vi "Insert Scheduled Transfer Handles.vi"(4 "Label in":T1 {"Words"."Param Setting"."Num Bits" min=1 max=32; "Words"."Param Setting"."Start Bit" min=8 max=31; "Words"."Block Data Refs"."Data Reference" format="%.0x"; "Label" format="%.0o"}, 7 "Tx channel handle in":u32, 8 "error in (no error)":errorcluster) -> (0 "error out":errorcluster, 3 "Label out":T1 {"Words"."Param Setting"."Num Bits" min=1 max=32; "Words"."Param Setting"."Start Bit" min=8 max=31; "Words"."Block Data Refs"."Data Reference" format="%.0x"; "Label" format="%.0o"})   [LabVIEW 2016, in "Ballard Arinc-429 Engine.lvlib"]
uses:
  Ballard Arinc-429 Engine.lvlib
  RT Controls/RT Label Settings.ctl
  Shared/Controls and Global/Label.ctl
  Shared/Controls and Global/transferPeriod.ctl
  RT Controls/Driver Data.ctl
  RT Controls/RT Word Settings.ctl
  <vilib>/NI Veristand/Custom Device API/Block Data Reference.ctl
  <vilib>/NI Veristand/Custom Device API/Data Reference.ctl
  RT Controls/RT Param Setting.ctl
  Shared/Controls and Global/Start Bit.ctl
  Shared/Controls and Global/Number of Bits.ctl
  Shared/Controls and Global/TransferType.ctl
  <instrlib>/AIT 429/AIT 429.lvlib
  Shared/Ballard Arinc-429 Shared.lvlib
  <vilib>/NI Veristand/Custom Device API/Custom Device API.lvlib
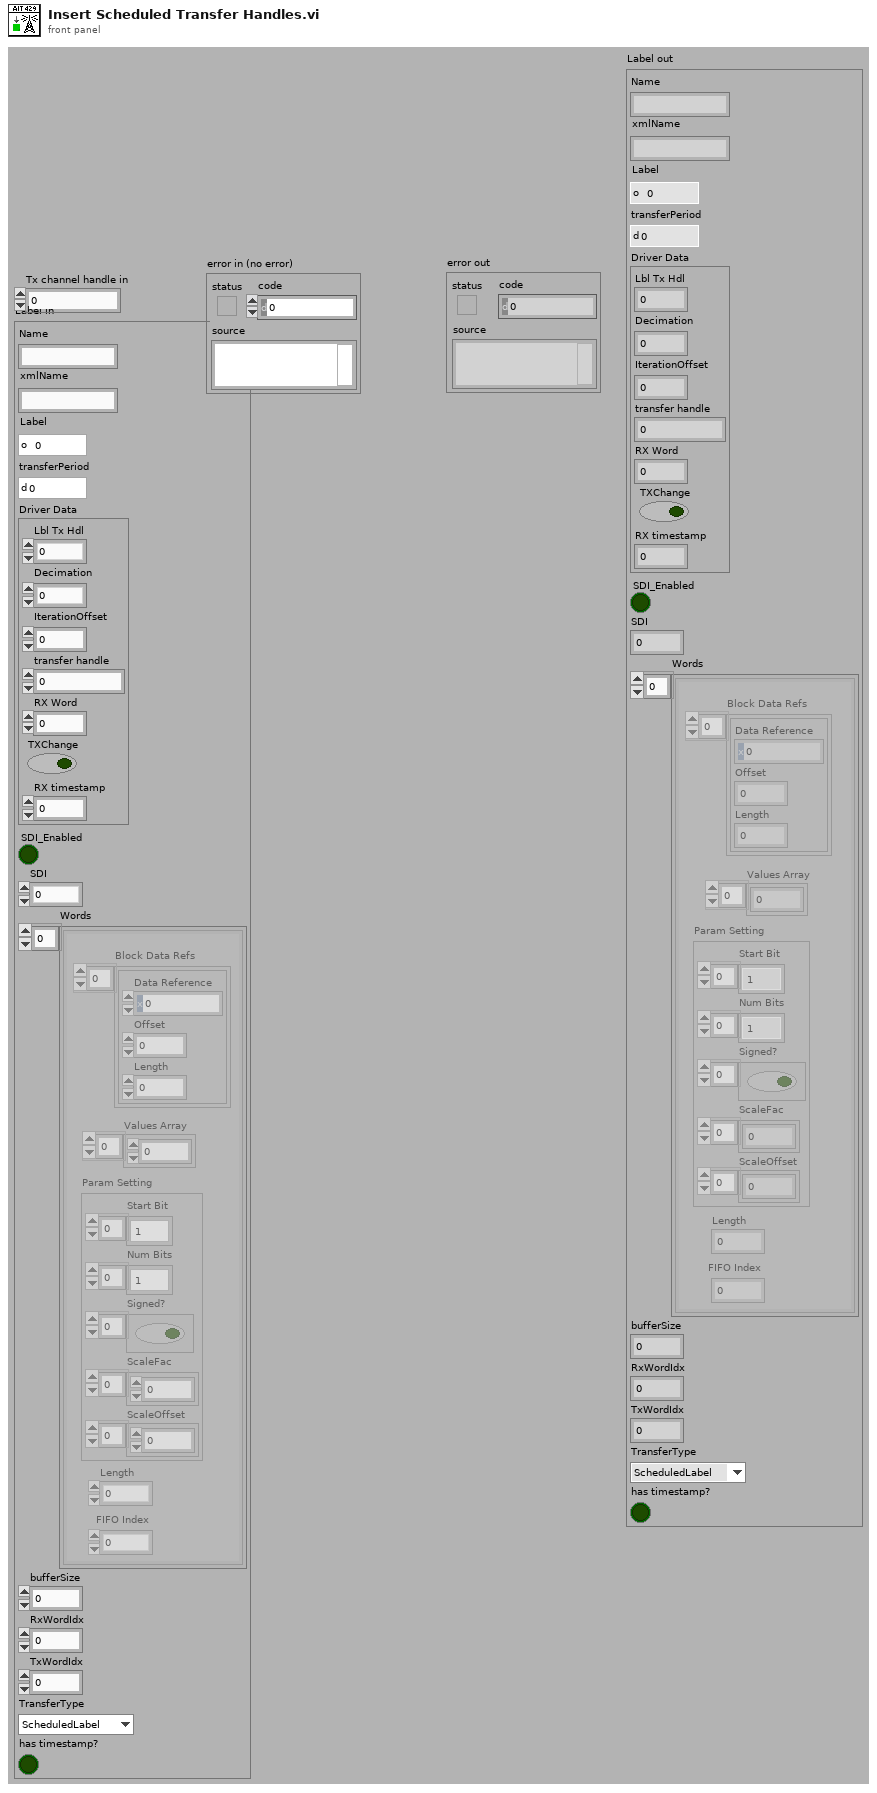
[diagram p1: front panel]
types:
  T1 = typedef "Ballard Arinc-429 Engine.lvlib/RT Label Settings.ctl" = cluster{"Name":string, "xmlName":string, "Label":T2, "transferPeriod":T3, "Driver Data":T4, "SDI_Enabled":bool, "SDI":u8, "Words":T5[], "bufferSize":u32, "RxWordIdx":i32, "TxWordIdx":i32, "TransferType":T11, "has timestamp?":bool}
  T2 = typedef "Ballard Arinc-429 Shared.lvlib/Label.ctl" = u8
  T3 = typedef "Ballard Arinc-429 Shared.lvlib/transferPeriod.ctl" = u32
  T4 = typedef "Ballard Arinc-429 Engine.lvlib/Driver Data.ctl" = cluster{"Lbl Tx Hdl":u32, "Decimation":i32, "IterationOffset":i32, "transfer handle":u32, "RX Word":u32, "TXChange":bool, "RX timestamp":dbl}
  T5 = typedef "Ballard Arinc-429 Engine.lvlib/RT Word Settings.ctl" = cluster{"Block Data Refs":T6[], "Values Array":dbl[], "Length":i32, "FIFO Index":i32, "Param Setting":T8}
  T6 = typedef "Custom Device API.lvlib/Block Data Reference.ctl" = cluster{"Data Reference":T7, "Offset":u64, "Length":u64}
  T7 = typedef "Custom Device API.lvlib/Data Reference.ctl" = i32
  T8 = typedef "Ballard Arinc-429 Engine.lvlib/RT Param Setting.ctl" = cluster{"Start Bit":T9[], "Num Bits":T10[], "Signed?":bool[], "ScaleFac":dbl[], "ScaleOffset":dbl[]}
  T9 = typedef "Ballard Arinc-429 Shared.lvlib/Start Bit.ctl" = i32
  T10 = typedef "Ballard Arinc-429 Shared.lvlib/Number of Bits.ctl" = i32
  T11 = typedef "Ballard Arinc-429 Shared.lvlib/TransferType.ctl" = enum16{"ScheduledLabel", "Acyclic", "Block", "Strobe"}
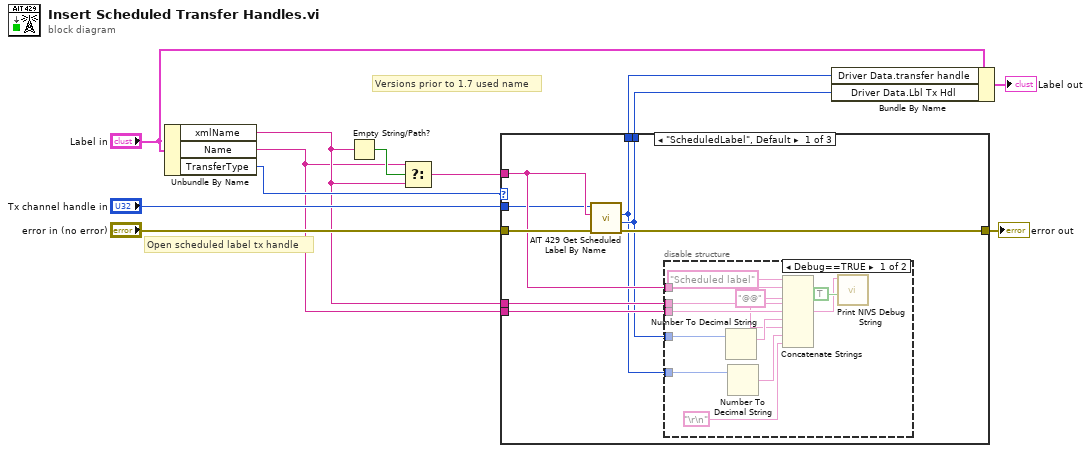
[diagram p0: block diagram]
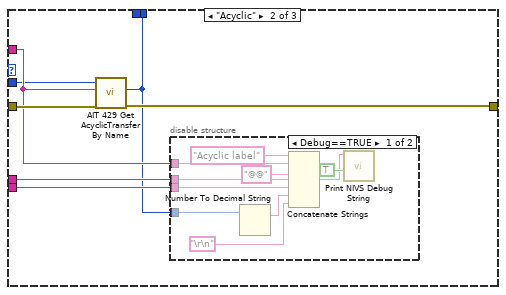
[diagram p3: hidden frame]
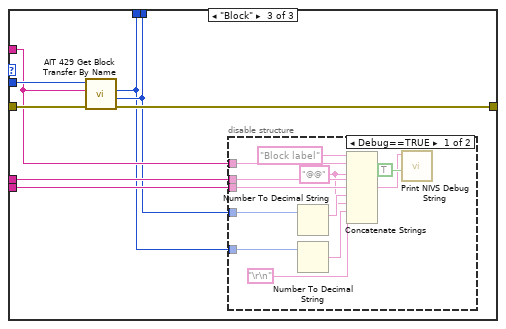
[diagram p5: hidden frame]
diagram:
  # "Open scheduled label tx handle"
  # "Versions prior to 1.7 used name"
  n1 = Unbundle By Name("Label in") -> ("xmlName"=w2:string, "Name"=w1:string, "TransferType"=w3:T11)
  n2 = Empty String/Path?(string/path=w2) -> (empty?=w5:bool)
  n3 = Select(t=w1, s=w5, f=w2) -> (s? t:f=w4:string)
  n4 = case shown="\"ScheduledLabel\", Default" w3 {
    tunnel: "error in (no error)" -> [w20 w39 w57]
    tunnel: [w14 w33 w51] -> w9
    tunnel: [w13 _ w50] -> w8
    tunnel: "Tx channel handle in" -> [w15 w34 w53]
    tunnel: [w19 w38 w56] -> w6
    tunnel: w4 -> [w18 w35 w52]
    tunnel: w2 -> [w17 w37 w55]
    tunnel: w1 -> [w16 w36 w54]
    frame "ScheduledLabel", Default {
      n5 = call <instrlib>:"AIT 429 Get Scheduled Label By Name.vi"("error in"=w20, "transfer name"=w18, "Tx channel handle in"=w15) -> ("error out"=w19:errorcluster, "scheduled label transfer handle out"=w14:u64, "rate oriented transfer handle out"=w13:u64)  [unwired: 3 in, 1 out]
      n6 = disable-structure shown="Debug==TRUE" {
        disable-tunnel: w18 -> [w29 _]
        disable-tunnel: w17 -> [w28 _]
        disable-tunnel: w16 -> [w27 _]
        disable-tunnel: w14 -> [w26 _]
        disable-tunnel: w13 -> [w22 _]
        frame condition #0 {
          w24 = "@@" ("string")
          n7 = Number To Decimal String(number=w26) -> (decimal integer string=w25:string)  [unwired: 1 in]
          n8 = Number To Decimal String(number=w22) -> (decimal integer string=w23:string)  [unwired: 1 in]
          n9 = Concatenate Strings("Scheduled label", w29, w24, w28, w27, w25, w24, w23, "\r\n") -> (w30:string)
          n10 = call "Print NIVS Debug String.vi"("Add to NIVS Log FIle? (T)"=TRUE, "Debug String"=w30) -> ()  [unwired: 8 in, 1 out]
        }
        frame condition #1 (active) {
        }
      }
    }
    frame "Acyclic" {
      n11 = call <instrlib>:"AIT 429 Get AcyclicTransfer By Name.vi"("error in"=w39, "transfer name"=w35, "channel handle"=w34) -> ("error out"=w38:errorcluster, "acyclic transfer handle out"=w33:u64)  [unwired: 6 in, 1 out]
      n12 = disable-structure shown="Debug==TRUE" {
        disable-tunnel: w35 -> [w46 _]
        disable-tunnel: w37 -> [w44 _]
        disable-tunnel: w36 -> [w43 _]
        disable-tunnel: w33 -> [w42 _]
        frame condition #0 {
          n13 = Number To Decimal String(number=w42) -> (decimal integer string=w41:string)  [unwired: 1 in]
          n14 = Concatenate Strings("Acyclic label", w46, "@@" ("string"), w44, w43, w41, "\r\n") -> (w47:string)
          n15 = call "Print NIVS Debug String.vi"("Add to NIVS Log FIle? (T)"=TRUE, "Debug String"=w47) -> ()  [unwired: 8 in, 1 out]
        }
        frame condition #1 (active) {
        }
      }
    }
    frame "Block" {
      n16 = call <instrlib>:"AIT 429 Get Block Transfer By Name.vi"("error in"=w57, "transfer name"=w52, "Tx channel handle in"=w53) -> ("error out"=w56:errorcluster, "block transfer handle out"=w51:u64, "rate oriented transfer handle out"=w50:u64)  [unwired: 3 in, 1 out]
      n17 = disable-structure shown="Debug==TRUE" {
        disable-tunnel: w52 -> [w66 _]
        disable-tunnel: w55 -> [w65 _]
        disable-tunnel: w54 -> [w64 _]
        disable-tunnel: w51 -> [w63 _]
        disable-tunnel: w50 -> [w60 _]
        frame condition #0 {
          w61 = "@@" ("string")
          n18 = Number To Decimal String(number=w63) -> (decimal integer string=w62:string)  [unwired: 1 in]
          n19 = Number To Decimal String(number=w60) -> (decimal integer string=w59:string)  [unwired: 1 in]
          n20 = Concatenate Strings("Block label", w66, w61, w65, w64, w62, w61, w59, "\r\n") -> (w67:string)
          n21 = call "Print NIVS Debug String.vi"("Add to NIVS Log FIle? (T)"=TRUE, "Debug String"=w67) -> ()  [unwired: 8 in, 1 out]
        }
        frame condition #1 (active) {
        }
      }
    }
  }
  "error out" <- w6
  n22 = Bundle By Name(cluster="Label in", "Driver Data.transfer handle"=w8, "Driver Data.Lbl Tx Hdl"=w9) -> (→"Label out":T1)
